vi "Read baudRate.vi"(8 "error in (no error)":errorcluster, 11 "OrionBMS in":refnum<class "Orion_BMS.lvclass">) -> (0 "error out":errorcluster, 2 "baudRate":u32(ring)=2 items=["1 Mbit/s"=0, "800 kbit/s"=1, "500 kbit/s"=2, "250 kbit/s"=3, "125 kbit/s"=4, "50 kbit/s"=6, "20 kbit/s"=7, "10 kbit/s"=8], 3 "OrionBMS out":refnum<class "Orion_BMS.lvclass">)   [LabVIEW 2018, in "Orion_BMS.lvclass"]
uses:
  Orion_BMS.lvclass
  Orion_BMS.lvclass/Orion_BMS.ctl
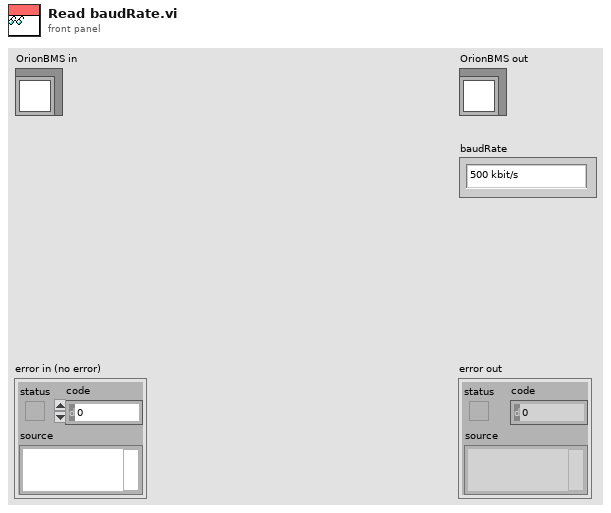
[diagram p1: front panel]
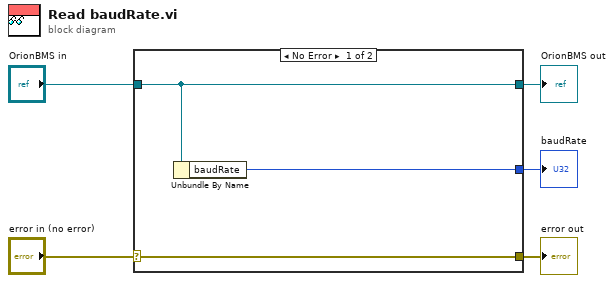
[diagram p0: block diagram]
diagram:
  n1 = case shown="No Error" "error in (no error)" {
    selector: "error in (no error)" -> [w8 w9]
    tunnel: [w8 w9] -> w4
    tunnel: [w7 w10] -> w2
    tunnel: "OrionBMS in" -> [w7 w10]
    tunnel: [w6 _] -> w1
    frame No Error {
      n2 = Unbundle By Name(w7) -> ("baudRate"=w6:u32)
    }
    frame Error {
    }
  }
  "error out" <- w4
  "OrionBMS out" <- w2
  "baudRate" <- w1
